vi "Configure Memory State.vi"(8 "error in (no error)":errorcluster, 9 "Auto Recall (F: Disable)":bool, 10 "Enable State Storage (F: Disable)":bool, 11 "VISA resource name":refnum<visa-resource-name>) -> (0 "error out":errorcluster, 3 "VISA resource name out":refnum<visa-resource-name>)   [LabVIEW 2020, in "Agilent 34405.lvlib"]
doc: "Configures the state storage settings of the instrument."
uses:
  <instrlib>/Agilent 34405/Agilent 34405.lvlib
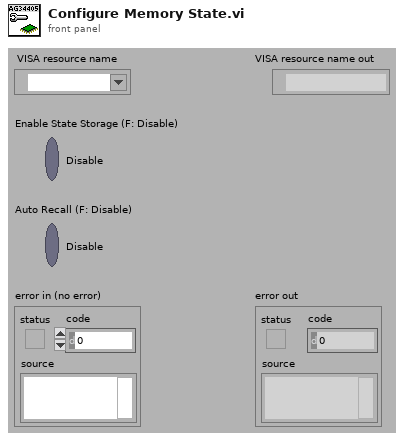
[diagram p1: front panel]
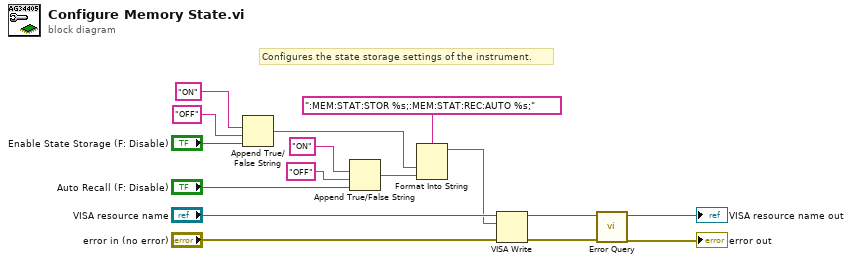
[diagram p0: block diagram]
diagram:
  # "Configures the state storage settings of the instrument."
  n1 = Append True/False String(1:"Enable State Storage (F: Disable)", 2:"OFF" ("false string"), 3:"ON" ("true string")) -> (0:w6:string)  [unwired: 1 out]
  n2 = Append True/False String(1:"Auto Recall (F: Disable)", 2:"OFF" ("false string"), 3:"ON" ("true string")) -> (0:w2:string)  [unwired: 1 out]
  n3 = Format Into String(format string=":MEM:STAT:STOR %s;:MEM:STAT:REC:AUTO %s;", w6, w2) -> (resulting string=w1:string)  [unwired: 2 in, 1 out]
  n4 = VISA Write(VISA resource name="VISA resource name", write buffer=w1, error in (no error)="error in (no error)") -> (VISA resource name out=w14:refnum<visa-resource-name>, error out=w13:errorcluster)  [unwired: 1 out]
  n5 = call <instrlib>:"Error Query.vi"("error in (no error)"=w13, "VISA resource name"=w14) -> ("error out"=→"error out":errorcluster, "VISA resource name out"=→"VISA resource name out":refnum<visa-resource-name>)  [unwired: 8 out]
